vi "Asyn Rx Ch FIFO State.vi"(9 "pState":u32, 10 "Channel":u8, 11 "devId":i32) -> (1 "pState out":u32, 2 "devId out":i32, 3 "function return":i32)   [LabVIEW 2013, in "CHR34XXX.lvlib"]
doc: "DLL BOOL __stdcall CHR34XXX_Asyn_RxCh_FIFOState(IN int devId,IN BYTE Channel,OUT DWORD *pState);"
uses:
  CHR34XXX.lvlib
  CHR34XXX.dll
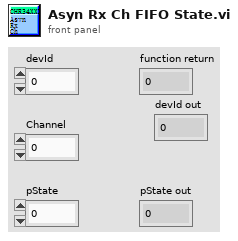
[diagram p1: front panel]
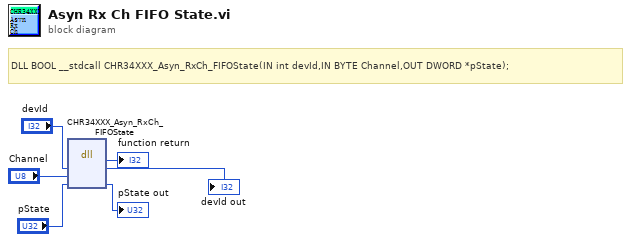
[diagram p0: block diagram]
diagram:
  # "DLL BOOL __stdcall CHR34XXX_Asyn_RxCh_FIFOState(IN int devId,IN BYTE Channel,OUT DWORD *pState);"
  n1 = dll-call lib="C:/Users/Administrator/Desktop/CHR34XXX_lv/lv_lib/CHR34XXX.*" fn="CHR34XXX_Asyn_RxCh_FIFOState"("devId"="devId", "Channel"="Channel", "pState"="pState") -> ("返回类型"=→"function return":i32, "devId"=→"devId out":i32, "pState"=→"pState out":u32)  [unwired: 4 in, 2 out]
